vi "gfitsio-create-tbl.vi"(4 "tbltype":T1 items=["ANY_HDU"=-1, "IMAGE_HDU"=0, "ASCII_TBL"=1, "BINARY_TBL"=2], 7 "extname":string, 8 "error in (no error)":errorcluster, 11 "gfits refnum":T2) -> (0 "error out":errorcluster, 3 "dup gfits refnum":T2)   [LabVIEW 2019, in "gfitsio.lvlib"]
doc: "Create a new ASCII or bintable table extension. The tbltype parameter defines the type of table and can have values of ASCII_TBL or BINARY_TBL. GFITSIO will automatically increase the size of the table as additional rows are written."
uses:
  gfitsio.lvlib
  gfitsio-refnum.ctl
  cfitsio-hdutypes.ctl
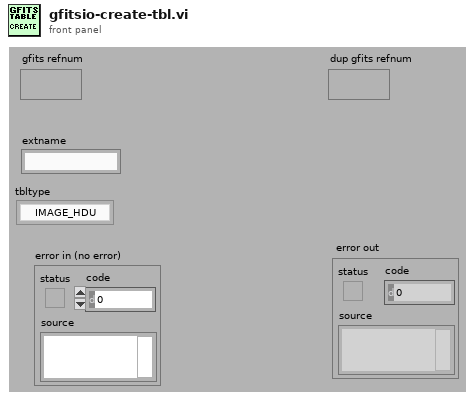
[diagram p1: front panel]
types:
  T1 = typedef "gfitsio.lvlib/cfitsio-hdutypes.ctl" = i32
  T2 = typedef "gfitsio.lvlib/gfitsio-refnum.ctl" = refnum<k1>
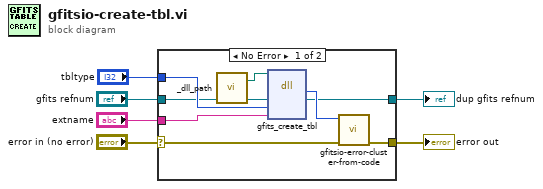
[diagram p0: block diagram]
diagram:
  n1 = case shown="No Error" "error in (no error)" {
    selector: "error in (no error)" -> [w12 w16]
    tunnel: [w14 w16] -> w6
    tunnel: "extname" -> [w11 _]
    tunnel: "gfits refnum" -> [w8 w15]
    tunnel: [w9 w15] -> w3
    tunnel: "tbltype" -> [w10 _]
    frame No Error {
      n2 = call "_dll_path.vi"() -> ("Path"=w7:path)  [unwired: 1 in]
      n3 = dll-call lib="?" fn="gfits_create_tbl"(path in=w7, "refnum"=w8, "tbltype"=w10, "extname"=w11) -> ("return type"=w13:i32, "refnum"=w9:T2)  [unwired: 4 in, 2 out]
      n4 = call "gfitsio-error-cluster-from-code.vi"("error in (no error)"=w12, "error code"=w13) -> ("error out"=w14:errorcluster)  [unwired: 9 out]
    }
    frame Error {
    }
  }
  "error out" <- w6
  "dup gfits refnum" <- w3
